vi "Database uploader.vi"() -> ()   [LabVIEW 2009]
uses:
  <vilib>/addons/database/Connection.llb/DB Tools Open Connec (Path).vi
  <vilib>/addons/database/NI_Database_API.lvlib
panel:
  in  "String 2":string="G"
  in  "String":string="76"
  out "data":variant[][](array[variant])
  out "columns":string[](array[string])
  out "error out":errorcluster
  out "tables":string[](array[string])
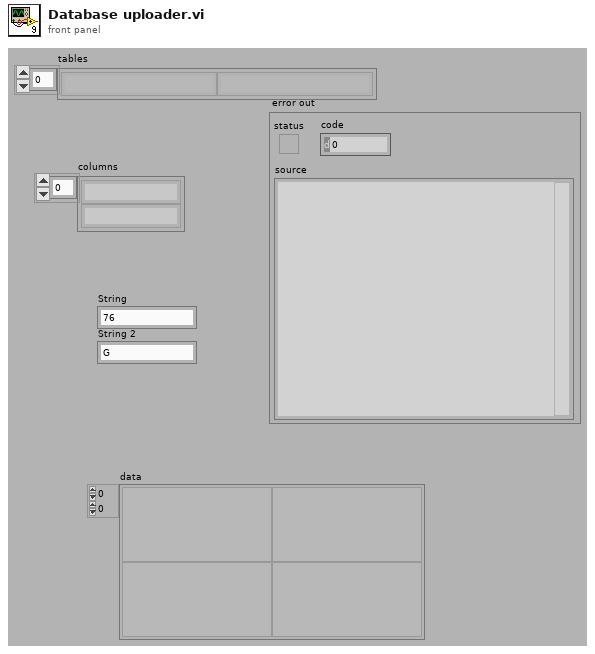
[diagram p1: front panel]
types:
  T1 = typedef "NI_Database_API.lvlib/Conn ObjectReference.ctl" = refnum<k1>
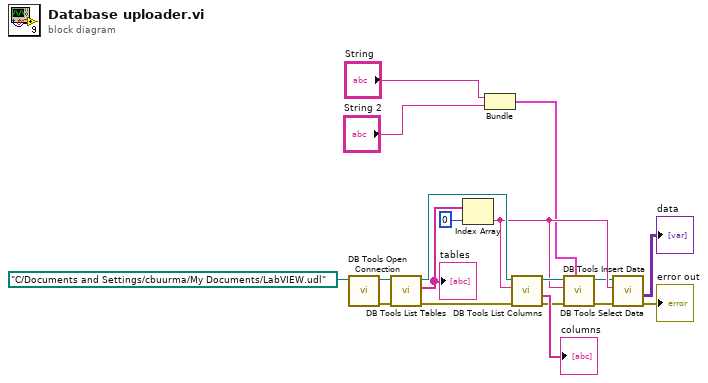
[diagram p0: block diagram]
diagram:
  n1 = call-poly <vilib>:"DB Tools Open Connection.vi"("connection information"=path "C:/Documents and Settings/cbuurma/My Documents/LabVIEW.udl") -> ("error out"=w17:errorcluster, "connection reference"=w16:T1)  [unwired: 7 in]
  n2 = call <vilib>:"DB Tools List Tables.vi"("error in (no error)"=w17, "connection reference"=w16) -> ("error out"=w12:errorcluster, "tables"=w15:string[], "connection reference out"=w13:T1)  [unwired: 3 in]
  "tables" <- w15
  n3 = Index Array(array=w15, index=0) -> (element=w8:string)
  n4 = Bundle("String"="String", "String 2"="String 2") -> (w3:cluster{"String":string, "String 2":string})  [unwired: 1 in]
  n5 = call <vilib>:"DB Tools List Columns.vi"("error in (no error)"=w12, "table"=w8, "connection reference"=w13) -> ("error out"=w9:errorcluster, "columns"=→"columns":string[], "connection reference out"=w11:T1)  [unwired: 1 in, 1 out]
  n6 = call <vilib>:"DB Tools Insert Data.vi"("data"=w3, "error in (no error)"=w9, "table"=w8, "connection reference"=w11) -> ("error out"=w5:errorcluster, "connection reference out"=w7:T1)  [unwired: 6 in]
  n7 = call <vilib>:"DB Tools Select Data.vi"("error in (no error)"=w5, "table"=w8, "connection reference"=w7) -> ("error out"=→"error out":errorcluster, "data"=→"data":variant[][])  [unwired: 3 in, 1 out]
